vi "USB - Read LineFeed Terminated String.vi"(8 "error in":errorcluster, 11 "VISA resource name in":refnum<visa-resource-name>) -> (0 "error out":errorcluster, 2 "Received Text":string, 3 "VISA resource name out":refnum<visa-resource-name>)   [LabVIEW 2021]
doc: "Read data from the USB/Serial connection, 1 byte at a time, until the newline character is encountered.\nThe newline character marks the end of the transmission."
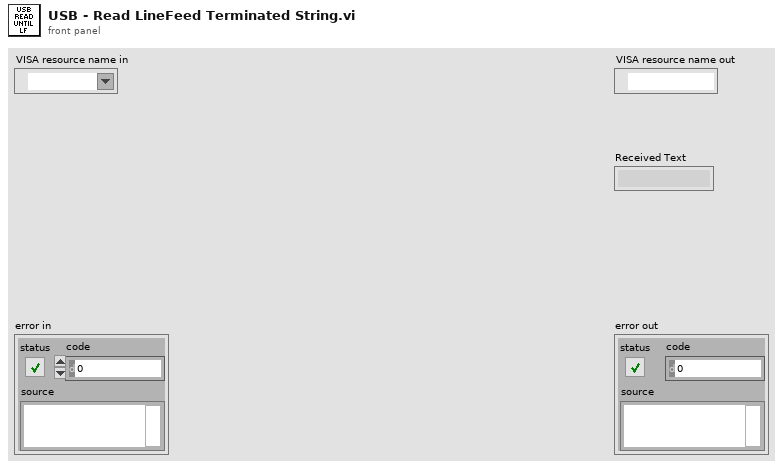
[diagram p1: front panel]
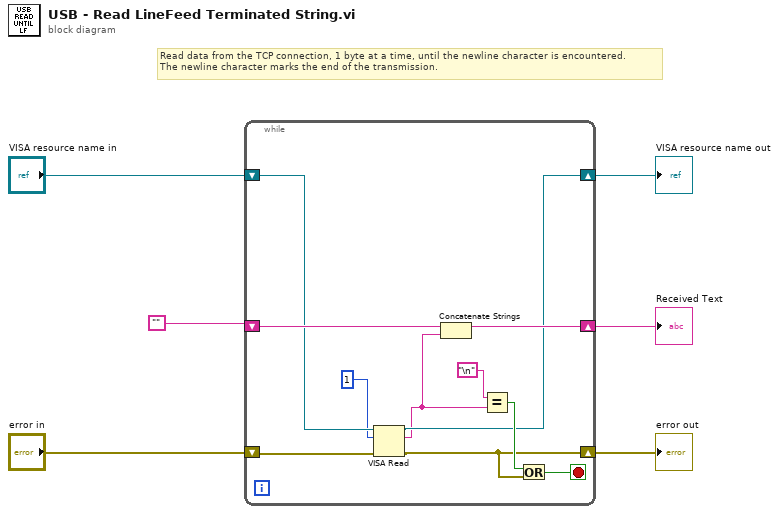
[diagram p0: block diagram]
diagram:
  # "Read data from the TCP connection, 1 byte at a time, until the newline character is encountered.\nThe newline character marks the end of the transmission."
  n1 = while {
    shift-right: [w11] -> w5
    shift-left: "error in" -> [w10]
    shift-right: [w12] -> w1
    shift-left: "VISA resource name in" -> [w9]
    shift-right: [w16] -> w3
    shift-left: "" -> [w17]
    stop <- w14 stop-if-true
    n2 = VISA Read(VISA resource name=w9, byte count=1 ("bytes to read"), error in (no error)=w10) -> (VISA resource name out=w12:refnum<visa-resource-name>, read buffer=w7:string, error out=w11:errorcluster)  [unwired: 1 out]
    n3 = Concatenate Strings(w17, w7) -> (w16:string)
    n4 = Equal?(x="\n", y=w7) -> (x = y?=w15:bool)
    n5 = Or(x=w15, y=w11) -> (x .or. y?=w14:bool)
  }
  "error out" <- w5
  "Received Text" <- w3
  "VISA resource name out" <- w1
